vi "BoolCmd_Recv.vi"(11 "Command Name":string) -> (0 "error out":errorcluster, 3 "New Request":bool)   [LabVIEW 2019, in "Trajectory_Library.lvlib"]
uses:
  Trajectory_Library.lvlib
  BoolCmd_ObtainQueue.vi
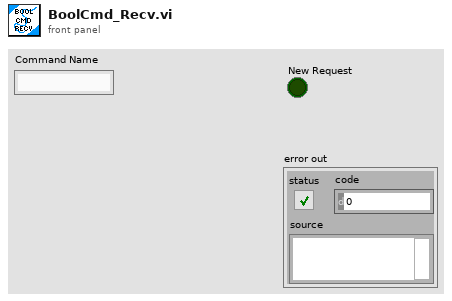
[diagram p1: front panel]
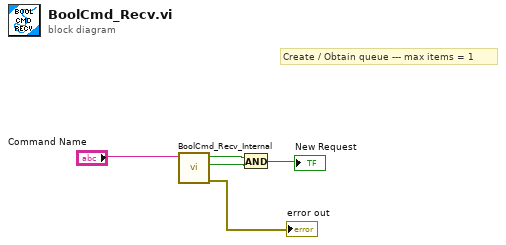
[diagram p0: block diagram]
diagram:
  # "Create / Obtain queue --- max items = 1"
  n1 = call "BoolCmd_Recv_Internal.vi"("Command Name"="Command Name") -> ("error out"=→"error out":errorcluster, "Newest Value"=w3:bool, "New Request"=w4:bool)  [unwired: 8 in]
  n2 = And(x=w4, y=w3) -> (x .and. y?=→"New Request":bool)
